vi "Pre Launch Init.vi"(11 "Watchdog in":refnum<class "Watchdog.lvclass">) -> (0 "error out":errorcluster, 3 "Watchdog out":refnum<class "Watchdog.lvclass">)   [LabVIEW 2015, in "Watchdog Actor.lvlib" / "Watchdog.lvclass"]
doc: "(<B>Filename</B>: Actor Framework.lvlib:Actor.lvclass:Pre Launch Init.vi)\n\nDefines behavior that occurs after the Launch Nested Actor method is invoked but before the actor's Actor Core method begins running.\n\nBy default, this method does nothing. A descendant class may override it to define behavior."
uses:
  Watchdog.lvclass
  Watchdog.lvclass/Watchdog.ctl
  <vilib>/ActorFramework/Actor/Actor.lvclass
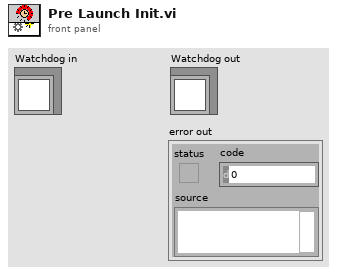
[diagram p1: front panel]
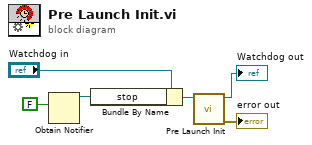
[diagram p0: block diagram]
diagram:
  n1 = Obtain Notifier(notification data type=FALSE) -> (notifier out=w3:refnum<notifier>)  [unwired: 3 in, 2 out]
  n2 = Bundle By Name(cluster="Watchdog in", "stop"=w3) -> (w1:refnum<class "Watchdog.lvclass">)
  n3 = call-parent "Pre Launch Init.vi"("Actor in"=w1) -> ("error out"=→"error out":errorcluster, "Actor out"=→"Watchdog out":refnum<class "Watchdog.lvclass">)  [unwired: 9 in]
